vi "parse_Foo.vi"(8 "error in":errorcluster, 11 "msg in":string) -> (0 "error out":errorcluster, 2 "Foo":cluster{" string1":string, " int1":u32}, 3 "msg out":string)   [LabVIEW 2015]
doc: "Parses a message into a foo"
uses:
  std_msgs/subs/parse_string_scalar.vi
  std_msgs/subs/parse_u32_scalar.vi
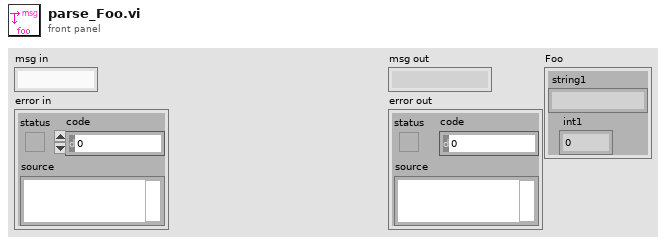
[diagram p1: front panel]
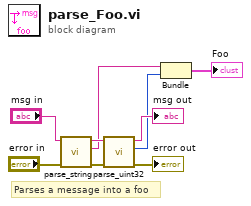
[diagram p0: block diagram]
diagram:
  # "Parses a message into a foo"
  n1 = call-poly "parse_string.vi"("error in"="error in", "msg in"="msg in") -> ("error out"=w6:errorcluster, "string"=w3:string, "msg out"=w7:string)  [unwired: 3 in]
  n2 = call-poly "parse_uint32.vi"("error in"=w6, "msg in"=w7) -> ("error out"=→"error out":errorcluster, "number"=w2:u32, "msg out"=→"msg out":string)  [unwired: 3 in]
  n3 = Bundle("string"=w3, "number"=w2) -> (→"Foo":cluster{"string":string, "number":u32})  [unwired: 1 in]
